vi "Rendezvous_2_a.vi"() -> ()   [LabVIEW 2019]
uses:
  <vilib>/Platform/TimedLoop/XDataNode/timing_clust.ctl
  <vilib>/Platform/TimedLoop/XDataNode/nitl_modes.ctl
  <vilib>/Platform/TimedLoop/XDataNode/wakeup.ctl
  <vilib>/Platform/TimedLoop/scheduler/LVUserAPI/_suppVIs/Create_1kHz_TSource.vi
  <vilib>/platform/TimedLoop/XDataNode/XDataNode.xnode
  <vilib>/Platform/TimedLoop/XDataNode/XDNodeRunTimeDep.lvlib
panel:
  out "Dioda":bool
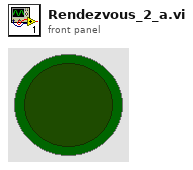
[diagram p1: front panel]
types:
  T1 = typedef "Rendezvous RefNum" = refnum<k1>
  T2 = typedef "XDNodeRunTimeDep.lvlib/timing_clust.ctl" = cluster{"Expected End [f-1]":u64, "Actual End [f-1]":u64, "Finished Late? [f-1]":bool, "Expected End [i-1]":u64, "Actual End [i-1]":u64, "Finished Late? [i-1]":bool, "Expected Start [i]":u64, "Actual Start [i]":u64, "Expected Start [f]":u64, "Actual Start [f]":u64, "Source Name":string, "Structure Name":string, "Period":i64, "Deadline":i64, "Offset":i64, "Start":i64, "Priority":i32, "Timeout":i32, "Mode":T3, "Wakeup Reason":T4, "Error":errorcluster, "Source Type":string, "Secondary Source Type":string, "Global End Time":u64, "Global Start Time":u64, "Frame Duration":u64, "Iteration Duration":u64, "Assigned CPU":i32, "I/O Scan Engine Mode":u32}
  T3 = typedef "XDNodeRunTimeDep.lvlib/nitl_modes.ctl" = enum32{"No Change", "Process missed periods, maintain original phase", "Discard missed periods, maintain original phase", "Process missed periods, ignore original phase", "Discard missed periods, ignore original phase"}
  T4 = typedef "XDNodeRunTimeDep.lvlib/wakeup.ctl" = enum32{"Normal", "Aborted", "Asynchronous wakeup", "Timing source error", "Timed loop error", "Timeout"}
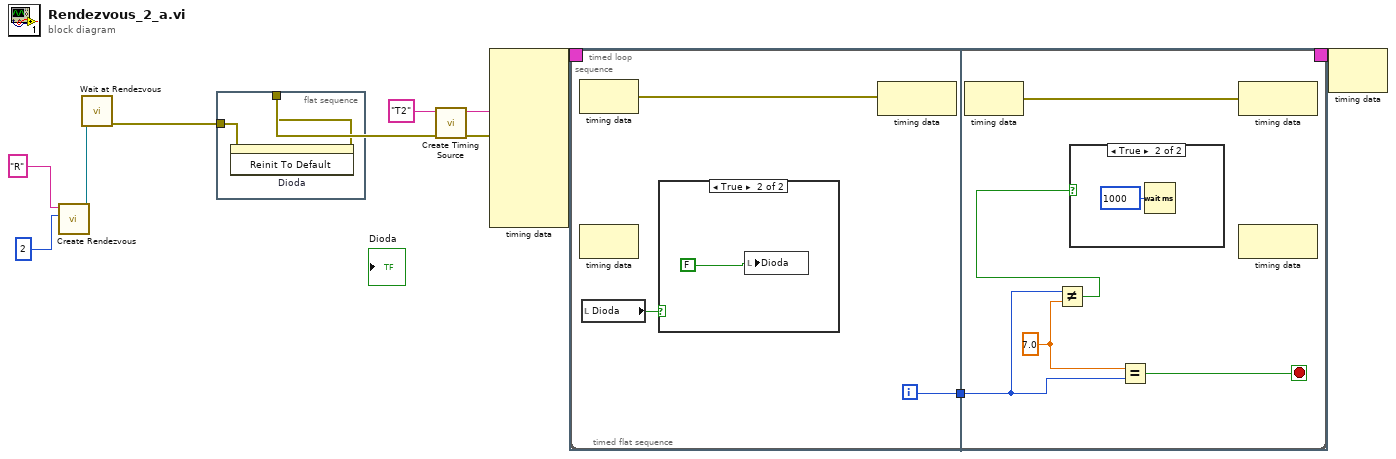
[diagram p0: block diagram]
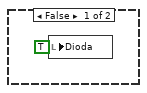
[diagram p2: hidden frame]
diagram:
  n1 = call <vilib>:"Create Rendezvous.vi"("size (2)"=2, "name (unnamed)"="R") -> ("rendezvous"=w3:T1)  [unwired: 3 in, 2 out]
  n2 = call <vilib>:"Wait at Rendezvous.vi"("rendezvous"=w3) -> ("error out"=w2:errorcluster)  [unwired: 4 in, 2 out]
  n3 = flat-sequence {
    tunnel: w2 -> [w12]
    tunnel: [w11] -> w1
    frame #0 {
      n4 = invoke on="Dioda" class="Bool (strict)" method="Reinit To Default"(error in=w12) -> (error out=w11:errorcluster)  [unwired: 2 in, 2 out]
    }
  }
  n5 = call-poly <vilib>:"Create Timing Source.vi"("error in (no error)"=w1, "name (in)"="T2") -> ("error out"=w7:errorcluster, "name (out)"=w8:string)  [unwired: 8 in]
  n6 = node-c288(w8, w7) -> (w10:T2)  [unwired: 8 in]
  n7 = timed-loop {
    timing: w10 -> [_]
    timing-out: [_] -> w9
    i -> [w14]
    stop <- w27 stop-if-true
    n8 = timed-sequence {
      timing: _ -> [_]
      timing-out: _ -> [_]
      n9 = timed-flat-sequence {
        tunnel: [w14] -> w13
        tunnel: w13 -> [w25]
        frame #0 {
          n10 = node-c288() -> (w16:errorcluster)  [unwired: 1 in]
          n11 = local read "Dioda"() -> (w15:bool)
          n12 = case shown="True" w15 {
            frame False {
              n13 = local write "Dioda"(TRUE ("LED")) -> ()
            }
            frame True {
              n14 = local write "Dioda"(FALSE ("LED")) -> ()
            }
          }
          n15 = node-c288(w16) -> ()  [unwired: 1 out]
        }
        frame #1 {
          w26 = 7.0 ("x")
          n16 = node-c288() -> (w28:errorcluster)  [unwired: 1 in]
          n17 = Not Equal?(x=w25, y=w26) -> (x != y?=w24:bool)
          n18 = case shown="True" w24 {
            frame False {
            }
            frame True {
              n19 = Wait (ms)(milliseconds to wait=u32 1000) -> ()  [unwired: 1 out]
            }
          }
          n20 = Equal?(x=w26, y=w25) -> (x = y?=w27:bool)
          n21 = node-c288(w28) -> ()  [unwired: 1 out]
        }
      }
    }
    n22 = node-c288() -> ()  [unwired: 1 in, 1 out]
    n23 = node-c288() -> ()  [unwired: 1 in, 1 out]
  }
  n24 = node-c288(w9) -> ()  [unwired: 1 out]
